vi "Median.vi"(10 "Rank":i32=15 min=1, 11 "Array in":dbl[](array[numeric])) -> (3 "Array out":dbl[](array[numeric]))   [LabVIEW 2013]
uses:
  <vilib>/Analysis/NI_AALBase.lvlib
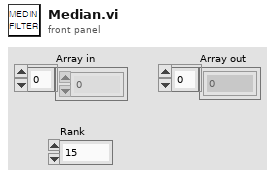
[diagram p1: front panel]
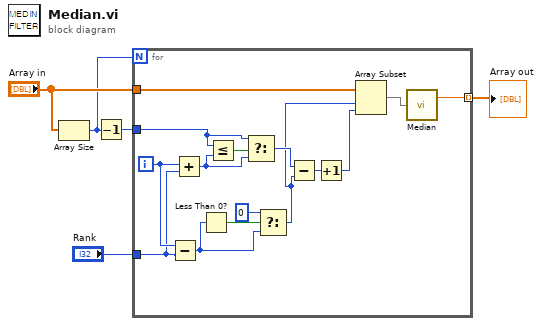
[diagram p0: block diagram]
diagram:
  n1 = Array Size(array="Array in") -> (size(s)=w2:i32)
  n2 = Decrement(x=w2) -> (x-1=w5:i32)
  n3 = for {
    N: w2 -> [_]
    tunnel: w5 -> [w14]
    tunnel: "Array in" -> [w10]
    tunnel: "Rank" -> [w16]
    tunnel: [w6] -> w1 mode=indexing
    i -> [w17]
    n4 = Subtract(x=w17, y=w16) -> (x-y=w18:i32)
    n5 = Add(x=w17, y=w16) -> (x+y=w13:i32)
    n6 = Less Than 0?(x=w18) -> (x < 0?=w19:bool)
    n7 = Less Or Equal?(x=w14, y=w13) -> (x <= y?=w15:bool)
    n8 = Select(t=w14, s=w15, f=w13) -> (s? t:f=w12:i32)
    n9 = Select(t=0, s=w19, f=w18) -> (s? t:f=w9:i32)
    n10 = Subtract(x=w12, y=w9) -> (x-y=w11:i32)
    n11 = Increment(x=w11) -> (x+1=w8:i32)
    n12 = Array Subset(array=w10, index=w9, length=w8) -> (w7:dbl[])
    n13 = call <vilib>:"Median.vi"("X"=w7) -> ("median"=w6:dbl)  [unwired: 1 out]
  }
  "Array out" <- w1
